vi "Axis_strings.vi"(1 "String":string) -> (0 "Enum":T1)   [LabVIEW 2010]
uses:
  Route mapping/Axis.ctl
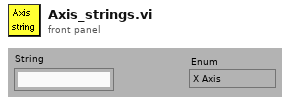
[diagram p1: front panel]
types:
  T1 = typedef "Axis.ctl" = enum16{"X Axis", "X Axis -ve", "Y Axis", "Y Axis -ve", "Z Axis", "Z Axis -ve"}
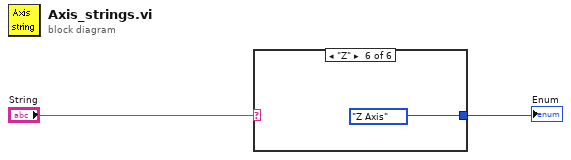
[diagram p0: block diagram]
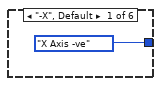
[diagram p2: hidden frame]
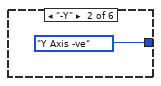
[diagram p3: hidden frame]
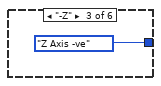
[diagram p4: hidden frame]
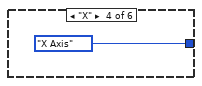
[diagram p5: hidden frame]
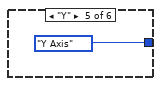
[diagram p6: hidden frame]
diagram:
  n1 = case shown="\"Z\"" "String" {
    tunnel: [Axis."X Axis -ve" ("Enum") Axis."Y Axis -ve" ("Enum") Axis."Z Axis -ve" ("Enum") Axis."X Axis" ("Enum") Axis."Y Axis" ("Enum") Axis."Z Axis" ("Enum")] -> w1
    frame "-X", Default {
    }
    frame "-Y" {
    }
    frame "-Z" {
    }
    frame "X" {
    }
    frame "Y" {
    }
    frame "Z" {
    }
  }
  "Enum" <- w1
